vi "axex_read_cells.vi"(7 "error proof read (True)":bool=TRUE, 8 "error in":errorcluster, 9 "right bottom cell":T1, 10 "top left cell":T1, 11 "AX Excel instance in":T2) -> (0 "error out":errorcluster, 1 "some cell is invalid?":bool, 2 "cell array":string[][](array[string]), 3 "AX Excel instance out":T2)   [LabVIEW 2020, in "AX Excel.lvlib"]
doc: "Call this to read array of cells. Array coordinates are given by top-left and bottom-right cell coordinates. The coordinates may be given as [column,row] index or cell name such as A1, AB66, ... with priority of cell name.\n\n'Error proof read' option means the VI will first try to read entire array at once as usually. If it fails it probably means some cell has invalid content so it will try to read the cells one by one so it should always return the array (with empty cells for the invalid cells). But keep in mind this can be painfully slow for larger arrays."
uses:
  AX Excel.lvlib
  axex_instance.ctl
  axex_cell_xy.ctl
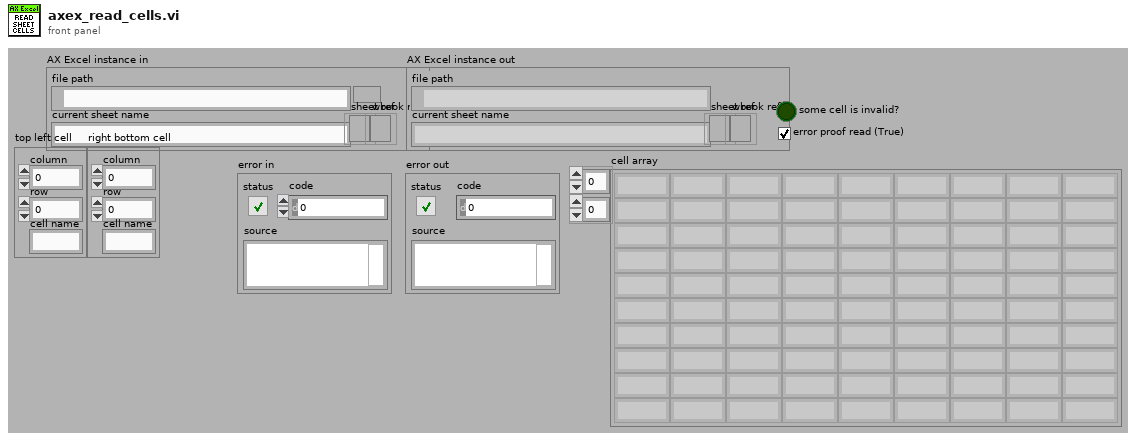
[diagram p1: front panel]
types:
  T1 = typedef "AX Excel.lvlib/axex_cell_xy.ctl" = cluster{"column":i32, "row":i32, "cell name":string}
  T2 = typedef "AX Excel.lvlib/axex_instance.ctl" = cluster{"file path":path, "current sheet name":string, "sheet ref":refnum<k7>, "wbook ref":refnum<k7>}
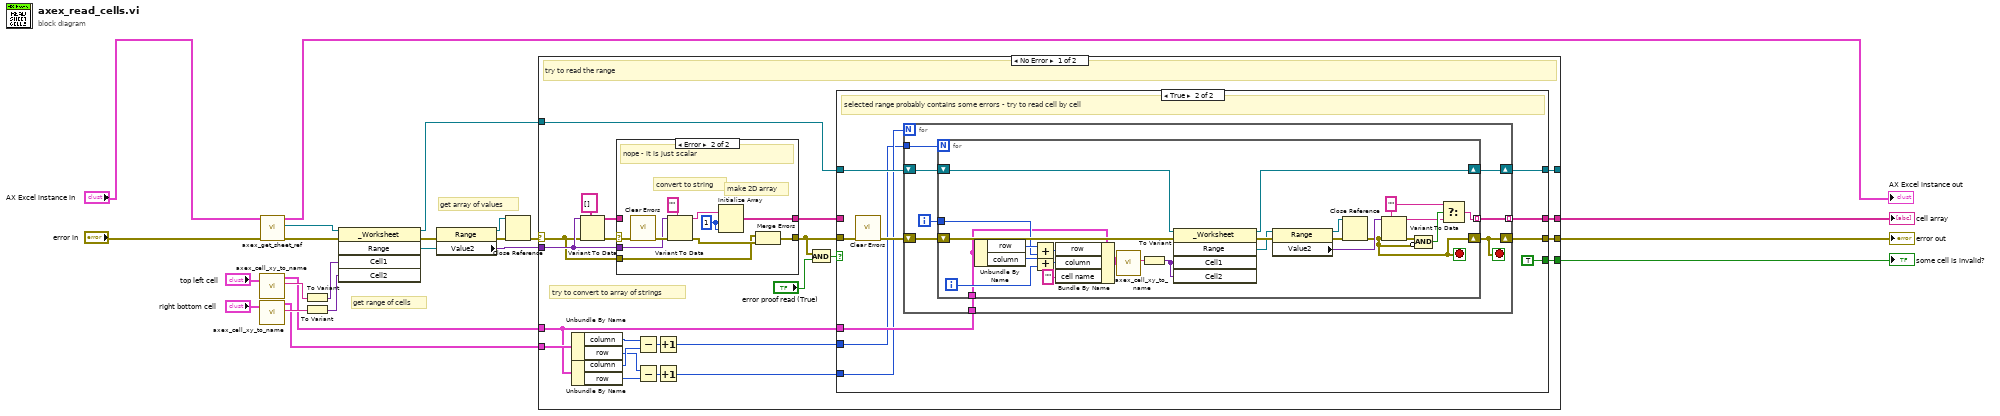
[diagram p0: block diagram]
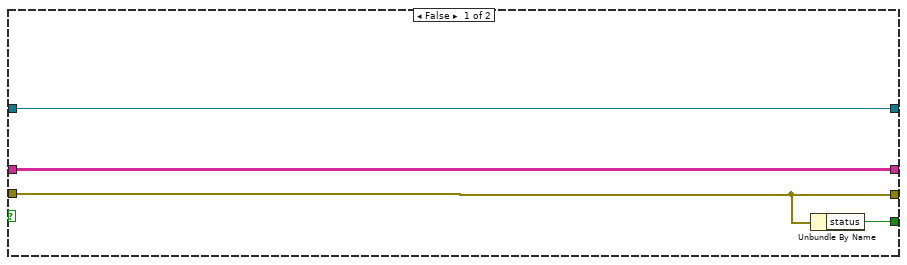
[diagram p2: hidden frame]
diagram:
  # "get array of values"
  # "get range of cells"
  n1 = call "axex_cell_xy_to_name.vi"("cell xy in"="top left cell") -> ("cell xy out"=w2:T1, "cell name"=w3:string)  [unwired: 1 in, 2 out]
  n2 = call "axex_cell_xy_to_name.vi"("cell xy in"="right bottom cell") -> ("cell xy out"=w1:T1, "cell name"=w10:string)  [unwired: 1 in, 2 out]
  n3 = call "axex_get_sheet_ref.vi"("error in"="error in", "AX Excel instance in"="AX Excel instance in") -> ("error out"=w14:errorcluster, "sheet ref out"=w17:refnum<k7>, "AX Excel instance out"=→"AX Excel instance out":T2)  [unwired: 6 in, 1 out]
  n4 = To Variant(anything=w3) -> (Variant=w16:variant)
  n5 = To Variant(anything=w10) -> (Variant=w15:variant)
  n6 = invoke class="_Worksheet" method="Range"(reference=w17, error in=w14, "Cell1"=w16, "Cell2"=w15) -> (reference out=w4:refnum<k7>, error out=w5:errorcluster, "Range"=w8:refnum<k7>)  [unwired: 1 in, 2 out]
  n7 = property class="Range"(reference=w8, error in=w5) -> (reference out=w12:refnum<k7>, error out=w13:errorcluster, "Value2"=w7:variant)
  n8 = Close Reference(reference=w12, error in (no error)=w13) -> (error out=w6:errorcluster)
  n9 = case shown="No Error" w6 {
    selector: w6 -> [w43 w108]
    tunnel: [w37 w108] -> w21
    tunnel: [w26 _] -> w22
    tunnel: w7 -> [w44 _]
    tunnel: w4 -> [w39 w107]
    tunnel: [w38 w107] -> _
    tunnel: w2 -> [w35 _]
    tunnel: w1 -> [w36 _]
    tunnel: [w24 _] -> w20
    frame No Error {
      # "try to convert to array of strings"
      # "try to read the range"
      n10 = Unbundle By Name(w36) -> ("column"=w34:i32, "row"=w31:i32)
      n11 = Unbundle By Name(w35) -> ("column"=w33:i32, "row"=w32:i32)
      n12 = Variant To Data(error in=w43, type=string[][] [], Variant=w44) -> (data=w45:string[][], error out=w46:errorcluster)
      n13 = case shown="Error" w46 {
        selector: w46 -> [w95 w99]
        tunnel: w44 -> [_ w97]
        tunnel: [w95 w100] -> w40
        tunnel: [w96 w103] -> w25
        tunnel: w45 -> [w96 _]
        tunnel: w43 -> [_ w98]
        frame No Error {
          # "is array so do nothing"
        }
        frame Error {
          w104 = 1 ("dimension size")
          # "make 2D array"
          # "convert to string"
          # "nope - it is just scalar"
          n14 = call <vilib>:"Clear Errors.vi"("error in (no error)"=w99) -> ("error out"=w102:errorcluster)  [unwired: 5 in, 1 out]
          n15 = Variant To Data(error in=w102, type="", Variant=w97) -> (data=w105:string, error out=w101:errorcluster)
          n16 = Initialize Array(w105, w104, w104) -> (w103:string[][])
          n17 = Merge Errors(w98, w101) -> (w100:errorcluster)
        }
      }
      n18 = Subtract(x=w34, y=w33) -> (x-y=w29:i32)
      n19 = Subtract(x=w31, y=w32) -> (x-y=w30:i32)
      n20 = Increment(x=w29) -> (x+1=w28:i32)
      n21 = Increment(x=w30) -> (x+1=w27:i32)
      n22 = Compound Arithmetic op=AND(w40, "error proof read (True)") -> (w41:bool)
      n23 = case shown="True" w41 {
        tunnel: w40 -> [w49 w56]
        tunnel: w39 -> [w51 w61]
        tunnel: [w51 w60] -> w38
        tunnel: [w49 w59] -> w37
        tunnel: w35 -> [_ w58]
        tunnel: w28 -> [_ w53]
        tunnel: w27 -> [_ w54]
        tunnel: [w50 w57] -> w26
        tunnel: w25 -> [w50 _]
        tunnel: [w48 TRUE] -> w24
        frame False {
          n24 = Unbundle By Name(w49) -> ("status"=w48:bool)
        }
        frame True {
          # "selected range probably contains some errors - try to read cell by cell"
          n25 = call <vilib>:"Clear Errors.vi"("error in (no error)"=w56) -> ("error out"=w55:errorcluster)  [unwired: 5 in, 1 out]
          n26 = for {
            N: w54 -> [_]
            shift-right: [w67] -> w60
            shift-left: w61 -> [w68]
            shift-right: [w63] -> w59
            shift-left: w55 -> [w69]
            tunnel: w58 -> [w66]
            tunnel: [w64] -> w57 mode=indexing
            tunnel: w53 -> [w62]
            i -> [w65]
            stop <- w63 stop-if-true
            n27 = for {
              N: w62 -> [_]
              shift-right: [w89] -> w67
              shift-left: w68 -> [w90]
              shift-right: [w71] -> w63
              shift-left: w69 -> [w94]
              tunnel: w66 -> [w82]
              tunnel: w65 -> [w83]
              tunnel: [w72] -> w64 mode=indexing
              i -> [w84]
              stop <- w71 stop-if-true
              w74 = ""
              n28 = Unbundle By Name(w82) -> ("row"=w88:i32, "column"=w85:i32)
              n29 = Add(x=w88, y=w83) -> (x+y=w87:i32)
              n30 = Add(x=w85, y=w84) -> (x+y=w86:i32)
              n31 = Bundle By Name(cluster=w82, "row"=w87, "column"=w86, "cell name"="") -> (w91:T1)
              n32 = call "axex_cell_xy_to_name.vi"("cell xy in"=w91) -> ("cell name"=w92:string)  [unwired: 1 in, 3 out]
              n33 = To Variant(anything=w92) -> (Variant=w93:variant)
              n34 = invoke class="_Worksheet" method="Range"(reference=w90, error in=w94, "Cell1"=w93, "Cell2"=w93) -> (reference out=w89:refnum<k7>, error out=w81:errorcluster, "Range"=w80:refnum<k7>)  [unwired: 1 in, 2 out]
              n35 = property class="Range"(reference=w80, error in=w81) -> (reference out=w78:refnum<k7>, error out=w79:errorcluster, "Value2"=w77:variant)
              n36 = Close Reference(reference=w78, error in (no error)=w79) -> (error out=w71:errorcluster)
              n37 = Variant To Data(error in=w71, type=w74, Variant=w77) -> (data=w73:string, error out=w76:errorcluster)
              n38 = Compound Arithmetic op=AND(w76, invert w71) -> (w75:bool)
              n39 = Select(t=w74, s=w75, f=w73) -> (s? t:f=w72:string)
            }
          }
        }
      }
    }
    frame Error {
      # "something fucked up seriously - do nothing"
    }
  }
  "error out" <- w21
  "cell array" <- w22
  "some cell is invalid?" <- w20
